vi "SetZLUT.vi"(1 "zlut":sgl[][](array[numeric]), 2 "profile_radius":sgl, 3 "tracker":u64) -> (0 "tracker":u64)   [LabVIEW 2011]
uses:
  TrackerDLL.vi
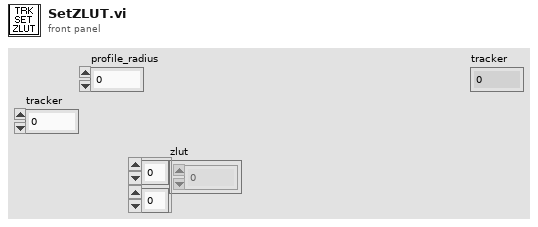
[diagram p1: front panel]
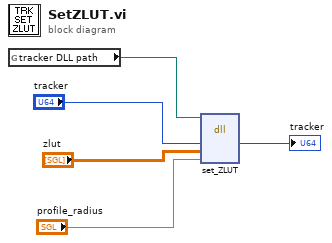
[diagram p0: block diagram]
diagram:
  n1 = global read "TrackerDLL.vi" "tracker DLL path"() -> (w5:path)
  n2 = dll-call lib="D:/jcnossen1/cudaqi-tracker/cudatrack-labview/cputrack_d.dll" fn="set_ZLUT"(path in=w5, "tracker"="tracker", "zlut"="zlut", "profile_radius"="profile_radius") -> ("tracker"=→"tracker":u64)  [unwired: 5 in, 2 out]
